vi "Open.vi"(8 "error in (no error)":errorcluster caption="entrée d'erreur (pas d'erreur)", 11 "Class CSV_File (Default) en entrée":refnum<class "Class File (Default).lvclass">) -> (0 "error out":errorcluster caption="sortie d'erreur", 3 "Class CSV_File (Default) en sortie":refnum<class "Class File (Default).lvclass">)   [LabVIEW 2020, in "Library Instrument & Equipement.lvlib" / "Library File.lvlib" / "Class File (Default).lvclass"]
uses:
  Class File (Default).lvclass
  Class File (Default).lvclass/Class File (Default).ctl
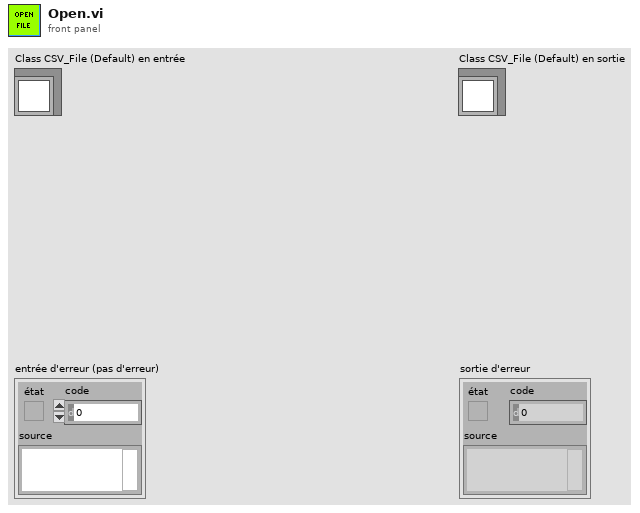
[diagram p1: front panel]
types:
  T1 = enum16{"open", "replace", "create", "open or create", "replace or create", "replace or create with confirmation"}
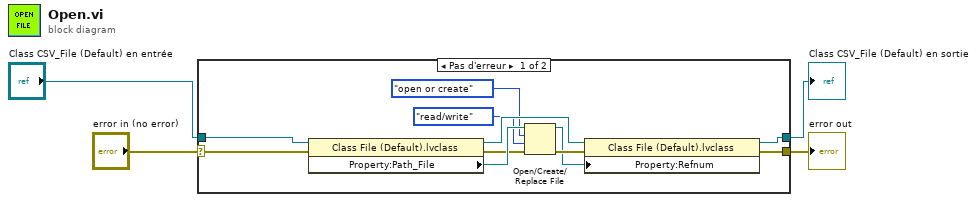
[diagram p0: block diagram]
diagram:
  n1 = case shown="Pas d'erreur" "error in (no error)" {
    selector: "error in (no error)" -> [w14 w17]
    tunnel: [w9 w17] -> w3
    tunnel: [w8 w16] -> w1
    tunnel: "Class CSV_File (Default) en entrée" -> [w12 w16]
    frame No Error {
      n2 = property class="Class File (Default).lvclass"(reference=w12, error in=w14) -> (reference out=w10:refnum<class "Class File (Default).lvclass">, error out=w13:errorcluster, "Property:Path_File"=w15:path)
      n3 = Open/Create/Replace File(file path (use dialog)=w15, error in=w13, operation (0:open)=T1."open or create" ("opération (0 : open)"), access (0:read/write)=enum16{"read/write", "read-only", "write-only"}."read/write" ("accès (0 : read/write)")) -> (refnum out=w7:refnum<file>, error out=w11:errorcluster)  [unwired: 2 in, 1 out]
      n4 = property class="Class File (Default).lvclass"(reference=w10, error in=w11, "Property:Refnum"=w7) -> (reference out=w8:refnum<class "Class File (Default).lvclass">, error out=w9:errorcluster)
    }
    frame Error {
    }
  }
  "error out" <- w3
  "Class CSV_File (Default) en sortie" <- w1
